vi "checkCallback.vi"(8 "error in (no error)":errorcluster, 11 "tcpServer in":refnum<class "TcpServer.lvclass">) -> (0 "error out":errorcluster, 2 "Packet":string, 3 "tcpServer out":refnum<class "TcpServer.lvclass">)   [LabVIEW 2018]
doc: "Receive a json packet from the Tcp Server and trigger an user event."
uses:
  TcpServer.lvclass
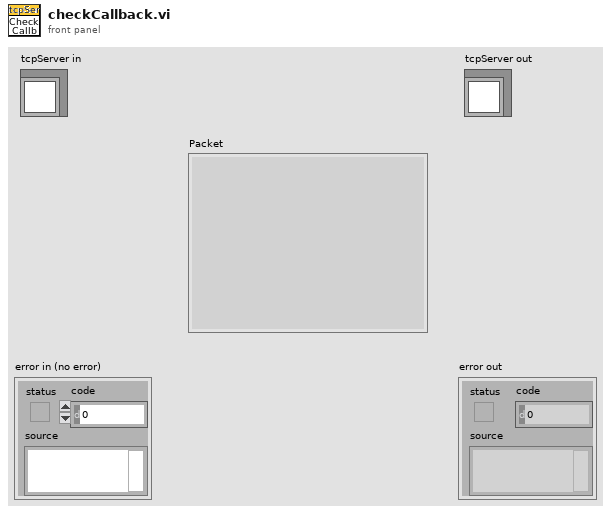
[diagram p1: front panel]
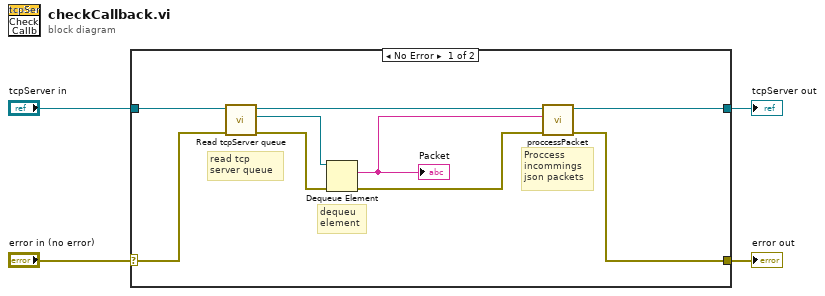
[diagram p0: block diagram]
diagram:
  n1 = case shown="No Error" "error in (no error)" {
    selector: "error in (no error)" -> [w12 w15]
    tunnel: [w5 w15] -> w3
    tunnel: [w8 w14] -> w1
    tunnel: "tcpServer in" -> [w13 w14]
    frame No Error {
      # "Proccess\nincommings\njson packets"
      # "dequeu\nelement"
      # "read tcp \nserver queue"
      n2 = call "Read tcpServer queue.vi"("error in (no error)"=w12, "tcpServer in"=w13) -> ("error out"=w10:errorcluster, "tcpServer queue"=w11:refnum<queue>, "tcpServer out"=w9:refnum<class "TcpServer.lvclass">)  [unwired: 7 in]
      n3 = Dequeue Element(queue=w11, error in (no error)=w10) -> (element=w7:string, error out=w6:errorcluster)  [unwired: 1 in, 2 out]
      "Packet" <- w7
      n4 = call "proccessPacket.vi"("error in (no error)"=w6, "tcp packet"=w7, "tcpServer in"=w9) -> ("error out"=w5:errorcluster, "tcpServer out"=w8:refnum<class "TcpServer.lvclass">)  [unwired: 7 in]
    }
    frame Error {
    }
  }
  "error out" <- w3
  "tcpServer out" <- w1
